vi "DQ_Multiplication.vi"(2 "DQ2":cluster{"q":T1, "qe":T1}, 3 "DQ1":cluster{"q":T1, "qe":T1}) -> (1 "Product":cluster{"q":T1, "qe":T1})   [LabVIEW 2014]
doc: "四元数的乘法"
uses:
  <vilib>/robotics/Kinematics/Quaternion.ctl
  <vilib>/robotics/Kinematics/Multiply Quaternion by Quaternion.vi
  <vilib>/robotics/Kinematics/NI_Kinematics.lvlib
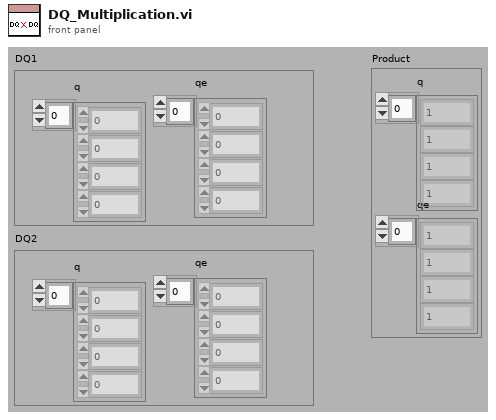
[diagram p1: front panel]
types:
  T1 = typedef "NI_Kinematics.lvlib/Quaternion.ctl" = dbl[]
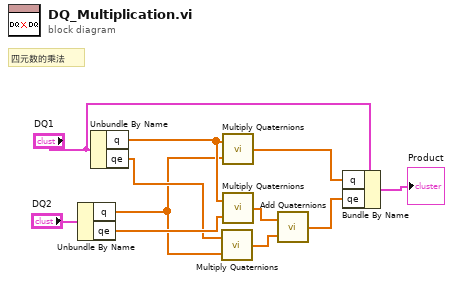
[diagram p0: block diagram]
diagram:
  # "四元数的乘法"
  n1 = Unbundle By Name("DQ2") -> ("q"=w7:T1, "qe"=w9:T1)
  n2 = Unbundle By Name("DQ1") -> ("q"=w10:T1, "qe"=w8:T1)
  n3 = call-poly <vilib>:"Multiply Quaternions.vi"("y"=w7, "quaternion"=w8) -> ("product"=w5:T1)
  n4 = call-poly <vilib>:"Multiply Quaternions.vi"("y"=w7, "quaternion"=w10) -> ("product"=w3:T1)
  n5 = call-poly <vilib>:"Multiply Quaternions.vi"("y"=w9, "quaternion"=w10) -> ("product"=w6:T1)
  n6 = call <vilib>:"Add Quaternions.vi"("quaternion 2"=w5, "quaternion 1"=w6) -> ("sum"=w2:T1)
  n7 = Bundle By Name(cluster="DQ1", "q"=w3, "qe"=w2) -> (→"Product":cluster{"q":T1, "qe":T1})
